vi "Configure Relative Offset.vi"(6 "Function (0: Volts)":u16(ring) items=["Volts", "Current", "Resistance", "Digitize Voltage", "Digitize Current"], 7 "Enable Releative Offset (T: Enable)":bool=TRUE, 8 "error in (no error)":errorcluster, 9 "Manual Offset (0)":dbl, 10 "Offset Mode (0: First Reading)":u16(ring) items=["First Reading", "Manual Offset"], 11 "VISA resource name":refnum<visa-resource-name>) -> (0 "error out":errorcluster, 3 "VISA resource name out":refnum<visa-resource-name>)   [LabVIEW 2018, in "Keithley 2450.lvlib"]
doc: "This command specifies the offset mode and relative offset value for the measurement."
uses:
  <instrlib>/Keithley 2450/Keithley 2450.lvlib
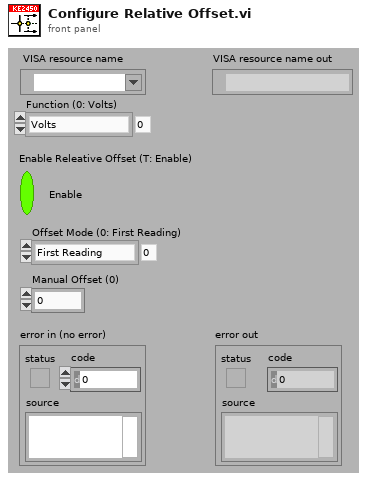
[diagram p1: front panel]
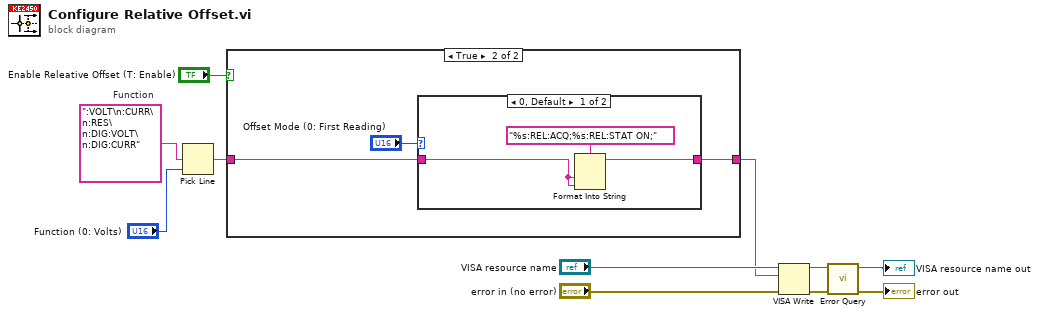
[diagram p0: block diagram]
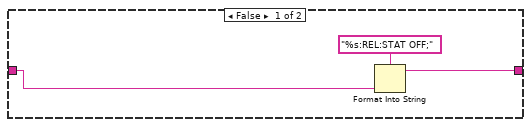
[diagram p2: hidden frame]
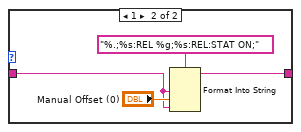
[diagram p3: hidden frame]
diagram:
  w3 = ":VOLT\n:CURR\n:RES\n:DIG:VOLT\n:DIG:CURR"  # Function
  n1 = Pick Line(multi-line string=w3, line index="Function (0: Volts)") -> (output string=w1:string)  [unwired: 1 out]
  n2 = case shown="True" "Enable Releative Offset (T: Enable)" {
    tunnel: [w14 w17] -> w5
    tunnel: w1 -> [w13 w15]
    frame False {
      n3 = Format Into String(format string="%s:REL:STAT OFF;", w13) -> (resulting string=w14:string)  [unwired: 2 in, 1 out]
    }
    frame True {
      n4 = case shown="0, Default" "Offset Mode (0: First Reading)" {
        tunnel: [w19 w24] -> w17
        tunnel: w15 -> [w18 w21]
        frame 0, Default {
          n5 = Format Into String(format string="%s:REL:ACQ;%s:REL:STAT ON;", w18, w18) -> (resulting string=w19:string)  [unwired: 2 in, 1 out]
        }
        frame 1 {
          n6 = Format Into String(format string="%.;%s:REL %g;%s:REL:STAT ON;", w21, "Manual Offset (0)", w21) -> (resulting string=w24:string)  [unwired: 2 in, 1 out]
        }
      }
    }
  }
  n7 = VISA Write(VISA resource name="VISA resource name", write buffer=w5, error in (no error)="error in (no error)") -> (VISA resource name out=w9:refnum<visa-resource-name>, error out=w6:errorcluster)  [unwired: 1 out]
  n8 = call <instrlib>:"Error Query.vi"("error in (no error)"=w6, "VISA resource name"=w9) -> ("error out"=→"error out":errorcluster, "VISA resource name out"=→"VISA resource name out":refnum<visa-resource-name>)  [unwired: 8 out]
